vi "readData.vi"(8 "error in (no error)":errorcluster, 9 "time readout loops [ms]":u32=500, 10 "Error String Out in":string, 11 "Channels":i32=6) -> (0 "error out":errorcluster, 2 "Error String Out out":string, 3 "Array":dbl[][](array[numeric]))   [LabVIEW 2021]
uses:
  <userlib>/er4commlib_labview/er4commlib_labview.lvlib
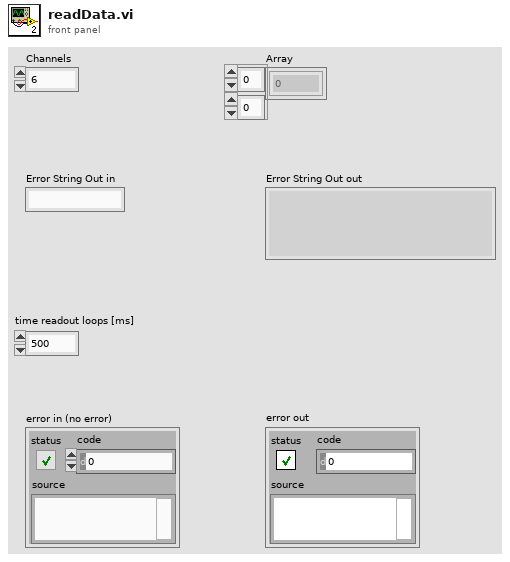
[diagram p1: front panel]
types:
  T1 = cluster{"availableDataPackets":u32, "bufferOverflowFlag":bool, "lostDataFlag":bool, "saturationFlag":bool, "currentRangeIncreaseFlag":bool, "currentRangeDecreaseFlag":bool, "communicationErrorFlag":bool}
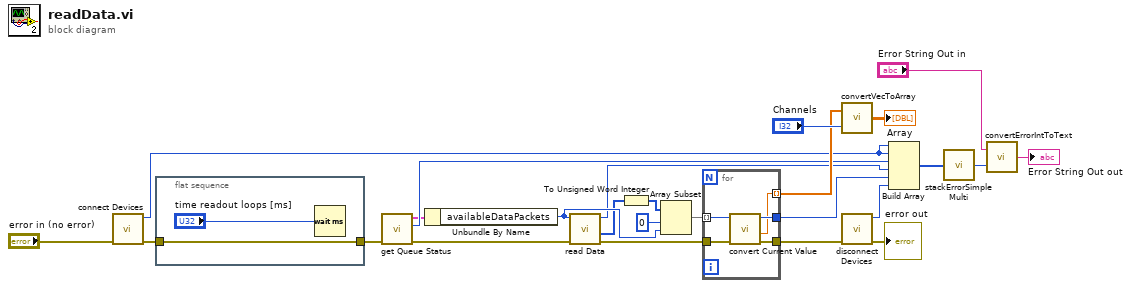
[diagram p0: block diagram]
diagram:
  n1 = call <userlib>:"connect Devices.vi"("error in (no error)"="error in (no error)") -> ("error out"=w16:errorcluster, "function return"=w17:u32)  [unwired: 9 in]
  n2 = flat-sequence {
    tunnel: w16 -> [w26]
    tunnel: [w26] -> w15
    frame #0 {
      n3 = Wait (ms)(milliseconds to wait="time readout loops [ms]") -> ()  [unwired: 1 out]
    }
  }
  n4 = call <userlib>:"get Queue Status.vi"("error in (no error)"=w15) -> ("error out"=w2:errorcluster, "function return"=w3:u32, "status out"=w1:T1)  [unwired: 8 in]
  n5 = Unbundle By Name(w1) -> ("availableDataPackets"=w22:u32)
  n6 = call <userlib>:"read Data.vi"("error in (no error)"=w2, "dataToRead"=w22) -> ("error out"=w8:errorcluster, "buffer out"=w14:i16[], "function return"=w4:u32)  [unwired: 6 in, 1 out]
  n7 = To Unsigned Word Integer(number=w14) -> (unsigned 16bit integer=w19:u16[])
  n8 = Array Subset(array=w19, index=0, length=w22) -> (w20:u16[])
  n9 = for {
    tunnel: w20 -> [w32] mode=indexing
    tunnel: [w28] -> w18 mode=indexing
    tunnel: [w31] -> w11
    tunnel: w8 -> [w30]
    tunnel: [w29] -> w9
    n10 = call <userlib>:"convert Current Value.vi"("error in (no error)"=w30, "intValue"=w32) -> ("error out"=w29:errorcluster, "fltValue out"=w28:dbl, "function return"=w31:u32)  [unwired: 7 in]
  }
  n11 = call "convertVecToArray.vi"("Channels"="Channels", "buffer in"=w18) -> ("Array"=→"Array":dbl[][])
  n12 = call <userlib>:"disconnect Devices.vi"("error in (no error)"=w9) -> ("error out"=→"error out":errorcluster, "function return"=w12:u32)  [unwired: 9 in]
  n13 = Build Array(w17, w17, w3, w4, w11, w12) -> (w5:u32[])
  n14 = call "stackErrorSimpleMulti.vi"("Error List"=w5) -> ("Error Out"=w6:u32)
  n15 = call "convertErrorIntToText.vi"("Error Int In (function return)"=w6, "Error String In"="Error String Out in") -> ("Error String Out"=→"Error String Out out":string)
